vi "Output_Config.vi"(0 "Drive Config":enum32{"Off", "On"}(radio), 1 "Right Motor":dbl, 2 "Left Motor":dbl, 3 "LED Config":u16(ring) items=["Off", "On"], 4 "Read_Config":i32[](array[numeric]), 5 "Motor Mode":enum32{"Coast", "Brake"}(radio), 6 "GPIO 1 Config":enum32{"Off", "Read", "Write", "PWM ", "Servo"}(radio), 7 "GPIO 2 Config":enum32{"Off", "Read", "Write", "PWM ", "Servo"}(radio), 8 "GPIO 3 Config":enum32{"Off", "Read", "Write", "PWM ", "Servo"}(radio), 9 "GPIO 1 Write":dbl, 10 "GPIO 2 Write":dbl, 13 "GPIO 3 Write":dbl, 14 "LINX Resource":T1, 15 "LED Write":bool, 16 "Error In":errorcluster) -> (17 "Error Out":errorcluster, 19 "LINX Resource":T1)   [LabVIEW 2016, in "ArgoBotLib.lvlib"]
uses:
  ArgoBotLib.lvlib
  <vilib>/MakerHub/LINX/Private/Type Defs/LINX Ref.ctl
  <vilib>/MakerHub/LINX/Private/Type Defs/Platform.ctl
  <vilib>/MakerHub/LINX/Private/Type Defs/Interface.ctl
  <vilib>/MakerHub/LINX/Private/Device/Type Defs/LINX Device Config.ctl
  <vilib>/MakerHub/LINX/Private/Device/Type Defs/TCP Config.ctl
  <vilib>/MakerHub/LINX/Private/Device/Type Defs/Channels.ctl
  <vilib>/MakerHub/LINX/Public/Peripherals/Digital/Digital Write N Chans.vi
  <vilib>/MakerHub/LINX/Private/Local IO/LinxDigitalWrite.vi
  <vilib>/MakerHub/LINX/Public/Utilities/Check Channel.vi
  <vilib>/MakerHub/LINX/Private/Utilties/Generate Error.vi
  <vilib>/MakerHub/LINX/Public/Peripherals/PWM/PWM Set Duty Cycle N Chans.vi
  <vilib>/MakerHub/LINX/Public/Sensors/Motion/Servo/Servo Set Pulse Width N Channels.vi
  <vilib>/MakerHub/LINX/LMH-LINX.lvlib
  <vilib>/MakerHub/LINX/Public/Sensors/Motion/Servo/Servo.lvlib
  <vilib>/MakerHub/LINX/Private/Device/Device.lvlib
panel:
  # "ArgoBot  Write Config"
  # "This vi writes and config the GPIO channels"
  # "Inputs"
  # "Outputs"
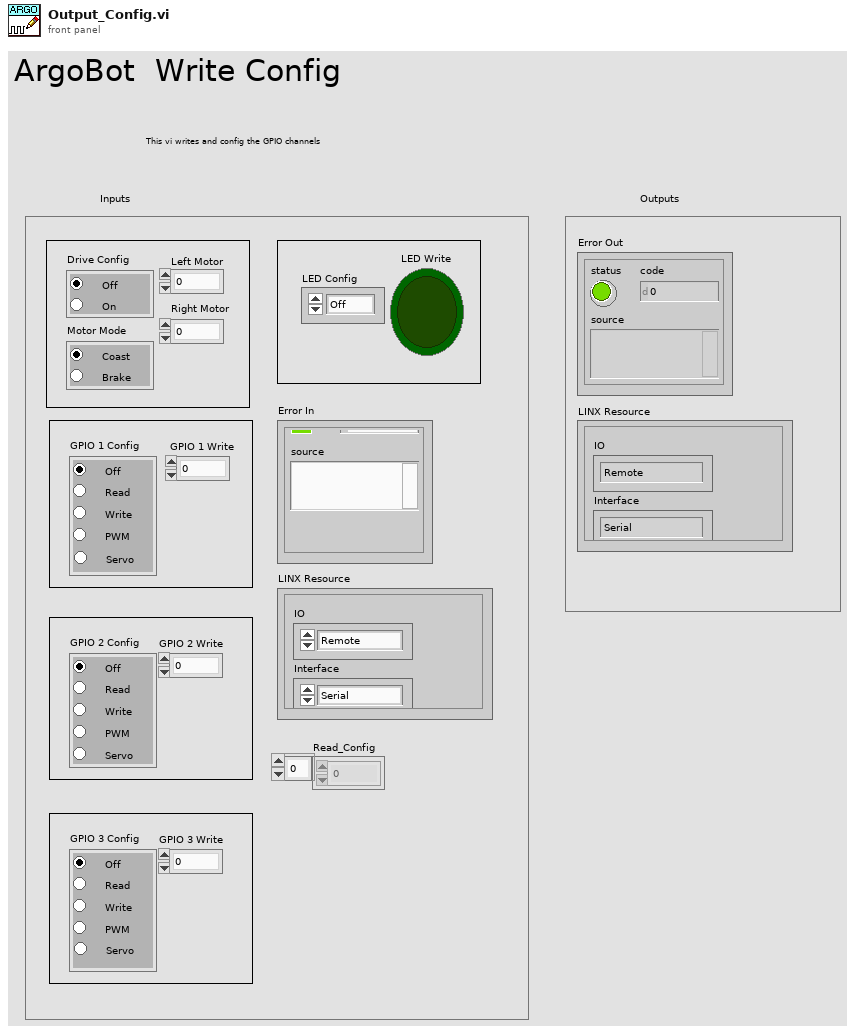
[diagram p1: front panel]
types:
  T1 = typedef "LMH-LINX.lvlib/LINX Ref.ctl" = cluster{"IO":T2, "Interface":T3, "LINX Device Config":T4}
  T2 = typedef "LMH-LINX.lvlib/Platform.ctl" = enum16{"Remote", "Local"}
  T3 = typedef "LMH-LINX.lvlib/Interface.ctl" = enum16{"Serial", "TCP"}
  T4 = typedef "LMH-LINX.lvlib/Device.lvlib/LINX Device Config.ctl" = cluster{"Interface":T3, "COM Port":refnum<visa-resource-name>, "TCP Configuration":T5, "Device Family":u8, "Device ID":u8, "Device Name":string, "TCP Ref":refnum<k5>, "Channels":T6}
  T5 = typedef "LMH-LINX.lvlib/Device.lvlib/TCP Config.ctl" = cluster{"IP Address":string, "Port":u16}
  T6 = typedef "LMH-LINX.lvlib/Channels.ctl" = cluster{"DI":u8[], "DO":u8[], "AI":u8[], "AO":u8[], "PWM":u8[], "QE":u8[], "UART":u8[], "I2C 2":u8[], "SPI":u8[], "CAN":u8[], "Servo":u8[], "AI Ref (V)":dbl, "AI Resolution (Bits)":u8, "AO Ref (V)":dbl, "AO Resolution (Bits)":u8}
  T7 = cluster{"Drive Config":enum32{"Off", "On"}, "Left Motor":dbl, "Right Motor":dbl, "GPIO 1 Config":enum32{"Off", "Read", "Write", "PWM ", "Servo"}, "GPIO 1 Write":dbl, "GPIO 2 Config":enum32{"Off", "Read", "Write", "PWM ", "Servo"}, "GPIO 2 Write":dbl, "GPIO 3 Config":enum32{"Off", "Read", "Write", "PWM ", "Servo"}, "GPIO 3 Write":dbl, "Error In":errorcluster, "LINX Resource":T1, "Read_Config":i32[], "Motor Mode":enum32{"Coast", "Brake"}, "LED Write":bool, "LED Config":u16}
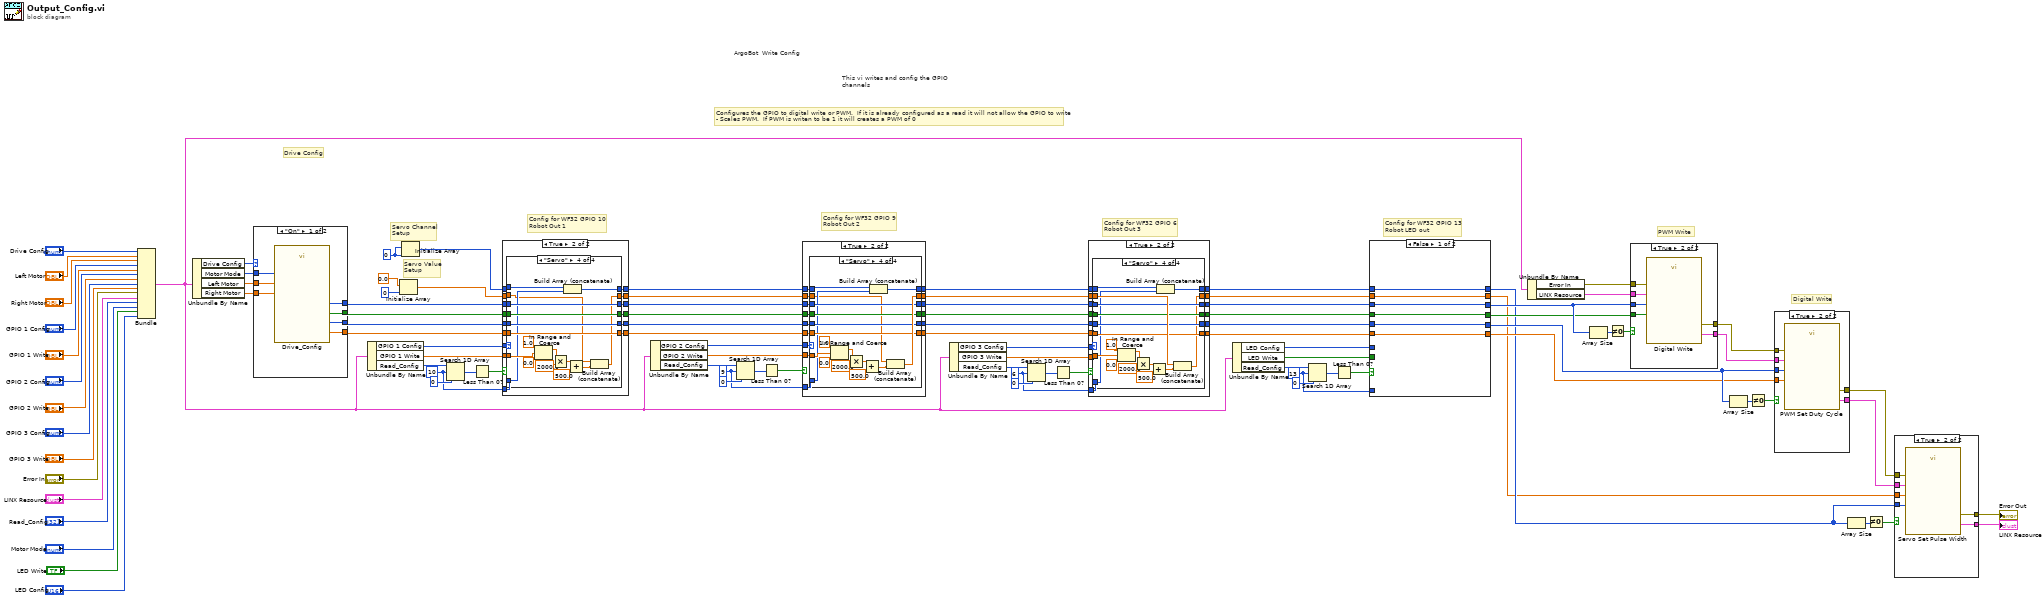
[diagram p0: block diagram]
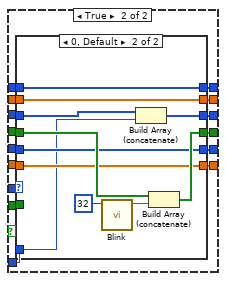
[diagram p3: hidden frame]
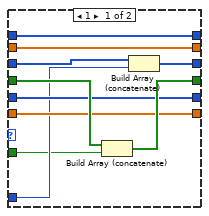
[diagram p4: hidden frame]
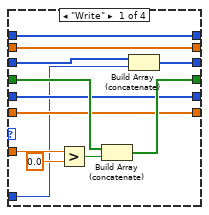
[diagram p6: hidden frame]
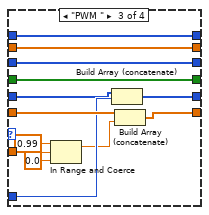
[diagram p8: hidden frame]
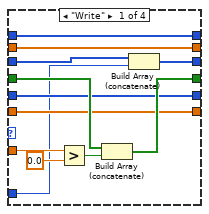
[diagram p10: hidden frame]
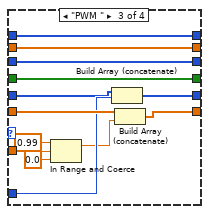
[diagram p12: hidden frame]
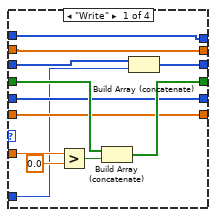
[diagram p14: hidden frame]
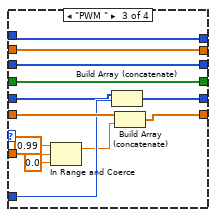
[diagram p16: hidden frame]
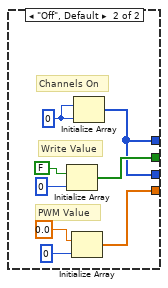
[diagram p19: hidden frame]
diagram:
  w16 = 0 ("dimension size")
  w30 = 13 ("element")
  w50 = 6 ("element")
  w52 = 9 ("element")
  w51 = 10 ("element")
  # "Servo Value\nSetup"
  # "Servo Channel\nSetup"
  # "Digital Write"
  # "PWM Write"
  # "Configures the GPIO to digital write or PWM.  If it is already configured as a read it will not allow the GPIO to write\n- Scales PWM.  If PWM is writen to be 1 it will creates a PWM of 0"
  # "This vi writes and config the GPIO channels"
  # "ArgoBot  Write Config"
  # "Config for WF32 GPIO 13\nRobot LED out"
  # "Config for WF32 GPIO 6\nRobot Out 3"
  # "Config for WF32 GPIO 9\nRobot Out 2"
  # "Config for WF32 GPIO 10\nRobot Out 1"
  # "Drive Config"
  n1 = Bundle("Drive Config"="Drive Config", "Left Motor"="Left Motor", "Right Motor"="Right Motor", "GPIO 1 Config"="GPIO 1 Config", "GPIO 1 Write"="GPIO 1 Write", "GPIO 2 Config"="GPIO 2 Config", "GPIO 2 Write"="GPIO 2 Write", "GPIO 3 Config"="GPIO 3 Config", "GPIO 3 Write"="GPIO 3 Write", "Error In"="Error In", "LINX Resource"="LINX Resource", "Read_Config"="Read_Config", "Motor Mode"="Motor Mode", "LED Write"="LED Write", "LED Config"="LED Config") -> (w21:T7)  [unwired: 1 in]
  n2 = Unbundle By Name(w21) -> ("Drive Config"=w40:enum32{"Off", "On"}, "Motor Mode"=w38:enum32{"Coast", "Brake"}, "Left Motor"=w95:dbl, "Right Motor"=w94:dbl)
  n3 = case shown="\"On\"" w40 {
    tunnel: w95 -> [w102 _]
    tunnel: w94 -> [w101 _]
    tunnel: [w100 w105] -> w92
    tunnel: [w99 w106] -> w91
    tunnel: [w98 w105] -> w90
    tunnel: [w97 w103] -> w89
    tunnel: w38 -> [w96 _]
    frame "On" {
      n4 = call "Drive_Config.vi"("Left_Power in"=w102, "Right_Power in"=w101, "Motor Mode"=w96) -> ("GPIO_Value"=w99:bool[], "PWM_Value"=w97:dbl[], "GPIO_Channels"=w100:u8[], "PWM Channels"=w98:u8[])  [unwired: 9 in]
    }
    frame "Off", Default {
      w110 = 0 ("dimension size")
      # "Channels On"
      # "Write Value"
      # "PWM Value"
      n5 = Initialize Array(FALSE, 0 ("dimension size")) -> (w106:bool[])
      n6 = Initialize Array(0.0, 0 ("dimension size")) -> (w103:dbl[])
      n7 = Initialize Array(w110, w110) -> (w105:i32[])
    }
  }
  n8 = Unbundle By Name(w21) -> ("GPIO 1 Config"=w93:enum32{"Off", "Read", "Write", "PWM ", "Servo"}, "GPIO 1 Write"=w88:dbl, "Read_Config"=w62:i32[])
  n9 = Initialize Array(0.0, 0 ("dimension size")) -> (w15:dbl[])
  n10 = Initialize Array(w16, w16) -> (w14:i32[])
  n11 = Search 1D Array(1D array=w62, element=w51, start index (0)=0) -> (index of element=w63:i32)
  n12 = Less Than 0?(x=w63) -> (x < 0?=w61:bool)
  n13 = case shown="True" w61 {
    tunnel: w93 -> [_ w131]
    tunnel: w92 -> [w116 w130]
    tunnel: w91 -> [w115 w129]
    tunnel: w90 -> [w114 w128]
    tunnel: w89 -> [w113 w127]
    tunnel: w88 -> [_ w126]
    tunnel: w51 -> [_ w125]
    tunnel: [w116 w124] -> w87
    tunnel: [w115 w123] -> w86
    tunnel: [w114 w122] -> w85
    tunnel: [w113 w121] -> w84
    tunnel: [w111 w120] -> w13
    tunnel: [w112 w119] -> w19
    tunnel: w15 -> [w111 w118]
    tunnel: w14 -> [w112 w117]
    frame False {
    }
    frame True {
      n14 = case shown="\"Servo\"" w131 {
        tunnel: w130 -> [w136 w149 w162 w179]
        tunnel: [w135 w149 w162 w179] -> w124
        tunnel: w129 -> [w140 w148 w161 w171]
        tunnel: [w139 w148 w161 w171] -> w123
        tunnel: w128 -> [w138 w147 w156 w170]
        tunnel: [w138 w147 w158 w170] -> w122
        tunnel: w127 -> [w137 w146 w160 w169]
        tunnel: [w137 w146 w159 w169] -> w121
        tunnel: w126 -> [w143 _ w155 w172]
        tunnel: w125 -> [w134 _ w157 w167]
        tunnel: [w132 w145 w151 w165] -> w120
        tunnel: [w133 w144 w150 w168] -> w119
        tunnel: w118 -> [w132 w145 w151 w163]
        tunnel: w117 -> [w133 w144 w150 w166]
        frame "Write" {
          n15 = Greater?(x=w143, y=0.0) -> (0:w141:bool)
          n16 = Build Array (concatenate)(w140, w141) -> (w139:bool[])
          n17 = Build Array (concatenate)(w136, w134) -> (w135:i32[])
        }
        frame "Off", Default {
        }
        frame "PWM " {
          n18 = In Range and Coerce(upper limit=0.99, x=w155, lower limit=0.0) -> (coerced(x)=w154:dbl)  [unwired: 1 out]
          n19 = Build Array (concatenate)(w156, w157) -> (w158:i32[])
          n20 = Build Array (concatenate)(w160, w154) -> (w159:dbl[])
        }
        frame "Servo" {
          n21 = In Range and Coerce(upper limit=1.0, x=w172, lower limit=0.0 ("upper limit")) -> (coerced(x)=w173:dbl)  [unwired: 1 out]
          n22 = Multiply(x=w173, y=2000.0) -> (x*y=w176:dbl)
          n23 = Build Array (concatenate)(w166, w167) -> (w168:i32[])
          n24 = Add(x=w176, y=500.0) -> (x+y=w164:dbl)
          n25 = Build Array (concatenate)(w163, w164) -> (w165:dbl[])
        }
      }
    }
  }
  n26 = Unbundle By Name(w21) -> ("GPIO 2 Config"=w83:enum32{"Off", "Read", "Write", "PWM ", "Servo"}, "GPIO 2 Write"=w82:dbl, "Read_Config"=w58:i32[])
  n27 = Search 1D Array(1D array=w58, element=w52, start index (0)=0) -> (index of element=w59:i32)
  n28 = Less Than 0?(x=w59) -> (x < 0?=w57:bool)
  n29 = case shown="True" w57 {
    tunnel: w87 -> [w185 w200]
    tunnel: w86 -> [w184 w199]
    tunnel: w85 -> [w183 w198]
    tunnel: w84 -> [w182 w197]
    tunnel: w83 -> [_ w196]
    tunnel: w82 -> [_ w195]
    tunnel: w52 -> [_ w194]
    tunnel: [w185 w193] -> w79
    tunnel: [w184 w192] -> w78
    tunnel: [w183 w191] -> w77
    tunnel: [w182 w190] -> w76
    tunnel: w19 -> [w181 w187]
    tunnel: w13 -> [w180 w189]
    tunnel: [w180 w188] -> w12
    tunnel: [w181 w186] -> w11
    frame False {
    }
    frame True {
      n30 = case shown="\"Servo\"" w196 {
        tunnel: w200 -> [w205 w218 w231 w236]
        tunnel: [w204 w218 w231 w236] -> w193
        tunnel: w199 -> [w209 w217 w230 w237]
        tunnel: [w208 w217 w230 w237] -> w192
        tunnel: w198 -> [w207 w216 w225 w238]
        tunnel: [w207 w216 w227 w238] -> w191
        tunnel: w197 -> [w206 w215 w229 w239]
        tunnel: [w206 w215 w228 w239] -> w190
        tunnel: w195 -> [w212 _ w224 w240]
        tunnel: w194 -> [w203 _ w226 w233]
        tunnel: w189 -> [w201 w213 w220 w232]
        tunnel: [w201 w213 w220 w241] -> w188
        tunnel: w187 -> [w202 w214 w219 w234]
        tunnel: [w202 w214 w219 w235] -> w186
        frame "Write" {
          n31 = Greater?(x=w212, y=0.0) -> (0:w210:bool)
          n32 = Build Array (concatenate)(w209, w210) -> (w208:bool[])
          n33 = Build Array (concatenate)(w205, w203) -> (w204:i32[])
        }
        frame "Off", Default {
        }
        frame "PWM " {
          n34 = In Range and Coerce(upper limit=0.99, x=w224, lower limit=0.0) -> (coerced(x)=w223:dbl)  [unwired: 1 out]
          n35 = Build Array (concatenate)(w225, w226) -> (w227:i32[])
          n36 = Build Array (concatenate)(w229, w223) -> (w228:dbl[])
        }
        frame "Servo" {
          n37 = In Range and Coerce(upper limit=1.0, x=w240, lower limit=0.0 ("upper limit")) -> (coerced(x)=w243:dbl)  [unwired: 1 out]
          n38 = Multiply(x=w243, y=2000.0) -> (x*y=w246:dbl)
          n39 = Add(x=w246, y=500.0) -> (x+y=w242:dbl)
          n40 = Build Array (concatenate)(w234, w233) -> (w235:i32[])
          n41 = Build Array (concatenate)(w232, w242) -> (w241:dbl[])
        }
      }
    }
  }
  n42 = Unbundle By Name(w21) -> ("GPIO 3 Config"=w81:enum32{"Off", "Read", "Write", "PWM ", "Servo"}, "GPIO 3 Write"=w80:dbl, "Read_Config"=w54:i32[])
  n43 = Search 1D Array(1D array=w54, element=w50, start index (0)=0) -> (index of element=w55:i32)
  n44 = Less Than 0?(x=w55) -> (x < 0?=w53:bool)
  n45 = case shown="True" w53 {
    tunnel: w81 -> [_ w269]
    tunnel: w80 -> [_ w268]
    tunnel: w79 -> [w254 w267]
    tunnel: w78 -> [w253 w266]
    tunnel: w77 -> [w252 w265]
    tunnel: w50 -> [_ w264]
    tunnel: w76 -> [w251 w263]
    tunnel: [w253 w262] -> w24
    tunnel: [w251 w261] -> w22
    tunnel: [w254 w260] -> w25
    tunnel: [w252 w259] -> w23
    tunnel: w12 -> [w249 w258]
    tunnel: w11 -> [w250 w255]
    tunnel: [w249 w257] -> w10
    tunnel: [w250 w256] -> w9
    frame False {
    }
    frame True {
      n46 = case shown="\"Servo\"" w269 {
        tunnel: w267 -> [w274 w287 w300 w305]
        tunnel: [w273 w287 w300 w305] -> w260
        tunnel: w266 -> [w278 w286 w299 w306]
        tunnel: [w277 w286 w299 w306] -> w262
        tunnel: w265 -> [w276 w285 w294 w307]
        tunnel: [w276 w285 w296 w307] -> w259
        tunnel: w263 -> [w275 w284 w298 w308]
        tunnel: [w275 w284 w297 w308] -> w261
        tunnel: w268 -> [w281 _ w293 w310]
        tunnel: w264 -> [w272 _ w295 w301]
        tunnel: w258 -> [w270 w282 w288 w309]
        tunnel: [w270 w282 w288 w304] -> w257
        tunnel: [w271 w283 w289 w303] -> w256
        tunnel: w255 -> [w271 w283 w289 w302]
        frame "Write" {
          n47 = Greater?(x=w281, y=0.0) -> (0:w279:bool)
          n48 = Build Array (concatenate)(w278, w279) -> (w277:bool[])
          n49 = Build Array (concatenate)(w274, w272) -> (w273:i32[])
        }
        frame "Off", Default {
        }
        frame "PWM " {
          n50 = In Range and Coerce(upper limit=0.99, x=w293, lower limit=0.0) -> (coerced(x)=w292:dbl)  [unwired: 1 out]
          n51 = Build Array (concatenate)(w294, w295) -> (w296:i32[])
          n52 = Build Array (concatenate)(w298, w292) -> (w297:dbl[])
        }
        frame "Servo" {
          n53 = In Range and Coerce(upper limit=1.0, x=w310, lower limit=0.0 ("upper limit")) -> (coerced(x)=w312:dbl)  [unwired: 1 out]
          n54 = Multiply(x=w312, y=2000.0) -> (x*y=w315:dbl)
          n55 = Add(x=w315, y=500.0) -> (x+y=w311:dbl)
          n56 = Build Array (concatenate)(w302, w301) -> (w303:i32[])
          n57 = Build Array (concatenate)(w309, w311) -> (w304:dbl[])
        }
      }
    }
  }
  n58 = Unbundle By Name(w21) -> ("LED Config"=w20:u16, "LED Write"=w35:bool, "Read_Config"=w32:i32[])
  n59 = Search 1D Array(1D array=w32, element=w30, start index (0)=0) -> (index of element=w33:i32)
  n60 = Less Than 0?(x=w33) -> (x < 0?=w31:bool)
  n61 = case shown="False" w31 {
    tunnel: w20 -> [_ w338]
    tunnel: w35 -> [_ w337]
    tunnel: w25 -> [w323 w336]
    tunnel: w24 -> [w322 w335]
    tunnel: w23 -> [w321 w334]
    tunnel: w30 -> [_ w333]
    tunnel: w22 -> [w320 w332]
    tunnel: [w322 w331] -> w28
    tunnel: [w320 w330] -> w26
    tunnel: [w323 w329] -> w29
    tunnel: [w321 w328] -> w27
    tunnel: w10 -> [w318 w327]
    tunnel: [w318 w326] -> w3
    tunnel: w9 -> [w319 w324]
    tunnel: [w319 w325] -> w4
    frame False {
    }
    frame True {
      n62 = case shown="0, Default" w338 {
        tunnel: w336 -> [w344 w355]
        tunnel: [w343 w354] -> w329
        tunnel: w335 -> [w348 w359]
        tunnel: [w347 w358] -> w331
        tunnel: w334 -> [w346 w357]
        tunnel: [w346 w357] -> w328
        tunnel: w332 -> [w345 w356]
        tunnel: [w345 w356] -> w330
        tunnel: w337 -> [w341 _]
        tunnel: w333 -> [w342 w353]
        tunnel: w327 -> [w339 w350]
        tunnel: [w339 w350] -> w326
        tunnel: [w340 w349] -> w325
        tunnel: w324 -> [w340 w349]
        frame 1 {
          n63 = Build Array (concatenate)(w348, w341) -> (w347:bool[])
          n64 = Build Array (concatenate)(w344, w342) -> (w343:i32[])
        }
        frame 0, Default {
          n65 = call "Blink.vi"("Blink_Rate (hz)"=32 ("Time_Limit")) -> ("Blink"=w352:bool)  [unwired: 10 in]
          n66 = Build Array (concatenate)(w355, w353) -> (w354:i32[])
          n67 = Build Array (concatenate)(w359, w352) -> (w358:bool[])
        }
      }
    }
  }
  n68 = Unbundle By Name(w21) -> ("Error In"=w73:errorcluster, "LINX Resource"=w72:T1)
  n69 = Array Size(array=w29) -> (size(s)=w69:i32)
  n70 = Not Equal To 0?(x=w69) -> (x != 0?=w68:bool)
  n71 = case shown="True" w68 {
    tunnel: [w361 w367] -> w75
    tunnel: [w360 w366] -> w74
    tunnel: w73 -> [w361 w365]
    tunnel: w72 -> [w360 w364]
    tunnel: w28 -> [_ w363]
    tunnel: w29 -> [_ w362]
    frame False {
    }
    frame True {
      n72 = call-poly <vilib>:"Digital Write.vi"("Error In"=w365, "Values"=w363, "DO Channels"=w362, "LINX Resource"=w364) -> ("Error Out"=w367:errorcluster, "LINX Resource"=w366:T1)  [unwired: 6 in]
    }
  }
  n73 = Array Size(array=w27) -> (size(s)=w67:i32)
  n74 = Not Equal To 0?(x=w67) -> (x != 0?=w66:bool)
  n75 = case shown="True" w66 {
    tunnel: w75 -> [w369 w371]
    tunnel: w74 -> [w368 w372]
    tunnel: [w369 w375] -> w8
    tunnel: [w368 w374] -> w7
    tunnel: w27 -> [_ w373]
    tunnel: w26 -> [_ w370]
    frame False {
    }
    frame True {
      n76 = call-poly <vilib>:"PWM Set Duty Cycle.vi"("Error In"=w371, "Duty Cycles"=w370, "PWM Channels"=w373, "LINX Resource"=w372) -> ("Error Out"=w375:errorcluster, "LINX Resource"=w374:T1)  [unwired: 6 in]
    }
  }
  n77 = Array Size(array=w4) -> (size(s)=w6:i32)
  n78 = Not Equal To 0?(x=w6) -> (x != 0?=w5:bool)
  n79 = case shown="True" w5 {
    tunnel: w8 -> [w377 w383]
    tunnel: w7 -> [w376 w382]
    tunnel: w4 -> [_ w381]
    tunnel: w3 -> [_ w380]
    tunnel: [w377 w379] -> w2
    tunnel: [w376 w378] -> w1
    frame False {
    }
    frame True {
      n80 = call-poly <vilib>:"Servo Set Pulse Width.vi"("Error In"=w383, "Pulse Widths (uS)"=w380, "Servo Channels"=w381, "LINX Resource"=w382) -> ("Error Out"=w379:errorcluster, "LINX Resource"=w378:T1)  [unwired: 6 in]
    }
  }
  "Error Out" <- w2
  "LINX Resource" <- w1
